vi "Apply Stamp.vi"(8 "error in":errorcluster, 9 "Slot Number":i32, 10 "Chuck Number":i32, 11 "GrabberTool in":refnum<class "GrabberTool Class.lvclass">) -> (0 "error out":errorcluster, 3 "GrabberTool out":refnum<class "GrabberTool Class.lvclass">)   [LabVIEW 2017, in "GrabberTool Class.lvclass"]
uses:
  GrabberTool Class.lvclass
  Config Manager Class/Type Definitions/Part Type.ctl
  Config Manager Class/Type Definitions/Offset.ctl
  WorkTable Class/WorkTable Class.lvclass
  Vec3d Class/Vec3d Class.lvclass
  Config Manager Class/Config Manager Class.lvclass
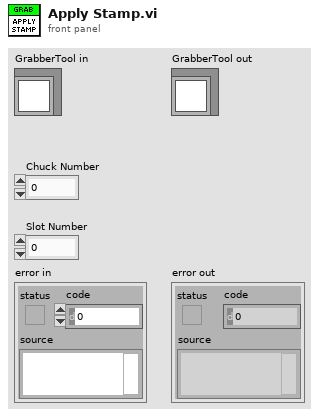
[diagram p1: front panel]
types:
  T1 = enum16{"Empty", "Bare HDI", "Unglued", "Stamped", "PartOnTop", "Weighted", "Unpotted", "Potted"}
  T2 = typedef "Offset.ctl" = enum16{"tool_holder_offset"}
  T3 = typedef "Part Type.ctl" = enum16{"BBM", "HDI", "BARE HDI", "GLUERESERVOIR", "STAMP_1", "STAMP_2", "STAMP_3", "STAMP_4", "STAMP_5", "STAMP_6", "STAMP_7", "STAMP_8", "WEIGHT_1", "WEIGHT_2", "WEIGHT_3", "WEIGHT_4", "WEIGHT_5", "WEIGHT_6", "WEIGHT_7", "WEIGHT_8", "WEIGHT_9", "WEIGHT_10", "WEIGHT_11", "WEIGHT_12", "WEIGHT_13", "WEIGHT_14", "WEIGHT_15", "WEIGHT_16", "PICKER_TOOL", "GRABER_TOOL"}
  T4 = typedef "Worktable_Module Slot.ctl" = cluster{"Slot State":enum16{"Empty", "Bare HDI", "Unglued", "Stamped", "PartOnTop", "Weighted", "Unpotted", "Potted"}, "BBM Type":enum16{"None", "BBM", "GlassSlide"}, "HDI Type":enum16{"None", "HDI", "Polyimide"}, "Vacuum Channel":u8, "Location/Orientation BBM":T5, "Location/Orientation HDI":T5, "S/N":string}
  T5 = typedef "Position_Orientation.ctl" = cluster{"Center":refnum<class "Vec3d Class.lvclass">, "Orientation":refnum<class "Orient3d Class.lvclass">}
  T6 = typedef "Stamp Type.ctl" = enum16{"Stamp 1", "Stamp 2", "Stamp 3", "Stamp 4", "Stamp 5", "Stamp 6", "Stamp 7", "Stamp 8"}
  T7 = typedef "Gluing Parameters.ctl" = cluster{"Safe Grabber Pickup":dbl, "Safe Grabber Lift":dbl, "Glue Resevoir Wait Time":dbl, "Glue BM Wait Time ":dbl, "Placed Weight X-Move":dbl}
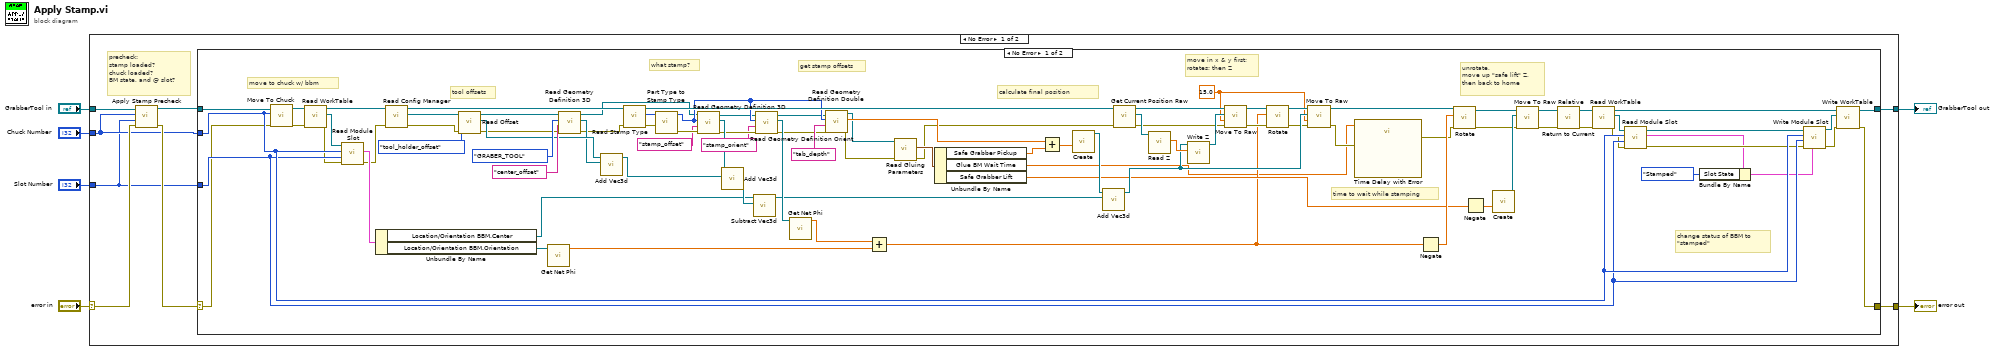
[diagram p0: block diagram]
diagram:
  n1 = case shown="No Error" "error in" {
    selector: "error in" -> [w10 w107]
    tunnel: [w14 w107] -> w6
    tunnel: "GrabberTool in" -> [w12 w108]
    tunnel: [w13 w108] -> w4
    tunnel: "Chuck Number" -> [w8 _]
    tunnel: "Slot Number" -> [w7 _]
    frame No Error {
      # "precheck:\nstamp loaded?\nchuck loaded?\nBM state, and @ slot?"
      n2 = call "Apply Stamp Precheck.vi"("error in (no error)"=w10, "Slot Number"=w7, "Chuck Number"=w8, "GrabberTool Class in"=w12) -> ("error out"=w9:errorcluster, "GrabberTool Class out"=w11:refnum<class "GrabberTool Class.lvclass">)  [unwired: 6 in]
      n3 = case shown="No Error" w9 {
        selector: w9 -> [w44 w106]
        tunnel: [w58 w106] -> w14
        tunnel: [w59 w105] -> w13
        tunnel: w11 -> [w104 w105]
        tunnel: w8 -> [w63 _]
        tunnel: w7 -> [w62 _]
        frame No Error {
          w42 = 15.0 ("Speed")
          # "move to chuck w/ bbm"
          # "time to wait while stamping"
          # "change status of BBM to\n\"stamped\""
          # "unrotate,\nmove up \"safe lift\" Z, \nthen back to home"
          # "move in x & y first;\nrotates; then Z"
          # "calculate final position"
          # "get stamp offsets"
          # "what stamp?"
          # "tool offsets"
          n4 = call-dynamic "Move To Chuck.vi"("error in"=w44, "Chuck"=w63, "Gantry in"=w104) -> ("error out"=w45:errorcluster, "Gantry out"=w101:refnum<class "GrabberTool Class.lvclass">)  [unwired: 7 in]
          n5 = call-dynamic "Read WorkTable.vi"("error in"=w45, "Gantry Class in"=w101) -> ("error out"=w46:errorcluster, "WorkTable Class.lvclass"=w100:refnum<class "WorkTable Class.lvclass">, "Gantry Class out"=w99:refnum<class "GrabberTool Class.lvclass">)  [unwired: 7 in]
          n6 = call-dynamic "Read Module Slot.vi"("error in"=w46, "slot"=w62, "chuck"=w63, "WorkTable in"=w100) -> ("error out"=w47:errorcluster, "Module Slot"=w103:T4)  [unwired: 5 in, 1 out]
          n7 = Unbundle By Name(w103) -> ("Location/Orientation BBM.Center"=w19:refnum<class "Vec3d Class.lvclass">, "Location/Orientation BBM.Orientation"=w89:refnum<class "Orient3d Class.lvclass">)
          n8 = call-dynamic "Read Config Manager.vi"("error in"=w47, "Gantry in"=w99) -> ("error out"=w48:errorcluster, "Config Manager"=w98:refnum<class "Config Manager Class.lvclass">, "Gantry out"=w94:refnum<class "GrabberTool Class.lvclass">)  [unwired: 7 in]
          n9 = call "Read Offset.vi"("error in"=w48, "Offset"=Offset."tool_holder_offset", "Config Manager in"=w98) -> ("error out"=w49:errorcluster, "Vec3d out"=w91:refnum<class "Vec3d Class.lvclass">, "Config Manager out"=w95:refnum<class "Config Manager Class.lvclass">)  [unwired: 6 in]
          n10 = call "Get Net Phi.vi"("Orient3d"=w89) -> ("phi(deg)"=w30:dbl)  [unwired: 8 in, 2 out]
          n11 = call "Read Geometry Definition 3D.vi"("error in"=w49, "Feature"="center_offset", "Part Type"=Part_Type."GRABER_TOOL", "Config Manager in"=w95) -> ("error out"=w50:errorcluster, "Feature Coordinates"=w90:refnum<class "Vec3d Class.lvclass">, "Config Manager out"=w36:refnum<class "Config Manager Class.lvclass">)  [unwired: 5 in]
          n12 = call-dynamic "Add Vec3d.vi"(10:"Vec3d Class in"=w90, 11:"Vec3d Class in"=w91) -> ("Vec3d Class out"=w22:refnum<class "Vec3d Class.lvclass">)  [unwired: 8 in, 1 out]
          n13 = call "Read Stamp Type.vi"("error in (no error)"=w50, "GrabberTool Class in"=w94) -> ("error out"=w51:errorcluster, "Stamp Type"=w93:T6, "GrabberTool Class out"=w83:refnum<class "GrabberTool Class.lvclass">)  [unwired: 7 in]
          n14 = call "Part Type to Stamp Type.vi"("error in"=w51, "Stamp Type"=w93) -> ("error out"=w28:errorcluster, "Part Type"=w37:T3)  [unwired: 8 in]
          n15 = call "Read Geometry Definition 3D.vi"("error in"=w28, "Feature"="stamp_offset", "Part Type"=w37, "Config Manager in"=w36) -> ("error out"=w27:errorcluster, "Feature Coordinates"=w33:refnum<class "Vec3d Class.lvclass">, "Config Manager out"=w35:refnum<class "Config Manager Class.lvclass">)  [unwired: 5 in]
          n16 = call-dynamic "Add Vec3d.vi"(10:"Vec3d Class in"=w22, 11:"Vec3d Class in"=w33) -> ("Vec3d Class out"=w20:refnum<class "Vec3d Class.lvclass">)  [unwired: 8 in, 1 out]
          n17 = call "Subtract Vec3d.vi"("Vec3d in 2"=w20, "Vec3d in 1"=w19) -> ("Vec3d Class out"=w21:refnum<class "Vec3d Class.lvclass">)  [unwired: 8 in, 1 out]
          n18 = call "Read Geometry Definition Orient.vi"("error in"=w27, "Feature"="stamp_orient", "Part Type"=w37, "Config Manager in"=w35) -> ("error out"=w24:errorcluster, "Orient3d out"=w32:refnum<class "Orient3d Class.lvclass">, "Config Manager out"=w34:refnum<class "Config Manager Class.lvclass">)  [unwired: 5 in]
          n19 = call "Get Net Phi.vi"("Orient3d"=w32) -> ("phi(deg)"=w29:dbl)  [unwired: 8 in, 2 out]
          n20 = call "Read Geometry Definition Double.vi"("error in"=w24, "Feature"="tab_depth", "Part Type"=w37, "Config Manager in"=w34) -> ("error out"=w38:errorcluster, "Geometry Definition"=w87:dbl, "Config Manager out"=w39:refnum<class "Config Manager Class.lvclass">)  [unwired: 5 in]
          n21 = Add(x=w29, y=w30) -> (x+y=w31:dbl)
          n22 = call "Read Gluing Parameters.vi"("error in (no error)"=w38, "Config Manager Class in"=w39) -> ("error out"=w52:errorcluster, "Gluing Parameters"=w102:T7)  [unwired: 7 in, 1 out]
          n23 = Unbundle By Name(w102) -> ("Safe Grabber Pickup"=w86:dbl, "Glue BM Wait Time"=w16:dbl, "Safe Grabber Lift"=w73:dbl)
          n24 = Add(x=w87, y=w86) -> (x+y=w85:dbl)
          n25 = call "Create.vi"("Z"=w85) -> ("Vec3d Class out"=w84:refnum<class "Vec3d Class.lvclass">)  [unwired: 9 in, 1 out]
          n26 = call-dynamic "Add Vec3d.vi"(10:"Vec3d Class in"=w21, 11:"Vec3d Class in"=w84) -> ("Vec3d Class out"=w76:refnum<class "Vec3d Class.lvclass">)  [unwired: 8 in, 1 out]
          n27 = call-dynamic "Get Current Position Raw.vi"("error in"=w52, "Gantry in"=w83) -> ("error out"=w23:errorcluster, "Vec3d Class out"=w81:refnum<class "Vec3d Class.lvclass">, "Gantry out"=w82:refnum<class "GrabberTool Class.lvclass">)  [unwired: 7 in]
          n28 = call-dynamic "Read Z.vi"("Vec3d Class in"=w81) -> ("Z"=w80:dbl)  [unwired: 8 in, 2 out]
          n29 = call-dynamic "Write Z.vi"("Z"=w80, "Vec3d Class in"=w76) -> ("Vec3d Class out"=w79:refnum<class "Vec3d Class.lvclass">)  [unwired: 8 in, 1 out]
          n30 = call-dynamic "Move To Raw.vi"("error in"=w23, "Speed"=w42, "Destination"=w79, "Gantry in"=w82) -> ("error out"=w53:errorcluster, "Gantry out"=w78:refnum<class "GrabberTool Class.lvclass">)  [unwired: 6 in]
          n31 = call-dynamic "Rotate.vi"("error in"=w53, "distance(deg)"=w31, "Gantry in"=w78) -> ("error out"=w54:errorcluster, "Gantry out"=w77:refnum<class "GrabberTool Class.lvclass">)  [unwired: 7 in]
          n32 = call-dynamic "Move To Raw.vi"("error in"=w54, "Speed"=w42, "Destination"=w76, "Gantry in"=w77) -> ("error out"=w17:errorcluster, "Gantry out"=w75:refnum<class "GrabberTool Class.lvclass">)  [unwired: 6 in]
          n33 = call "Time Delay with Error.vi"("error in (no error)"=w17, "Delay Time (s)"=w16) -> ("error out"=w15:errorcluster)  [unwired: 9 in]
          n34 = Negate(x=w31) -> (-x=w74:dbl)
          n35 = call-dynamic "Rotate.vi"("error in"=w15, "distance(deg)"=w74, "Gantry in"=w75) -> ("error out"=w69:errorcluster, "Gantry out"=w70:refnum<class "GrabberTool Class.lvclass">)  [unwired: 7 in]
          n36 = Negate(x=w73) -> (-x=w72:dbl)
          n37 = call "Create.vi"("Z"=w72) -> ("Vec3d Class out"=w71:refnum<class "Vec3d Class.lvclass">)  [unwired: 9 in, 1 out]
          n38 = call-dynamic "Move To Raw Relative.vi"("error in"=w69, "Delta"=w71, "Gantry in"=w70) -> ("error out"=w67:errorcluster, "Gantry out"=w68:refnum<class "GrabberTool Class.lvclass">)  [unwired: 7 in]
          n39 = call-dynamic "Return to Current.vi"("error in"=w67, "Gantry in"=w68) -> ("error out"=w65:errorcluster, "Gantry out"=w66:refnum<class "GrabberTool Class.lvclass">)  [unwired: 8 in]
          n40 = call-dynamic "Read WorkTable.vi"("error in"=w65, "Gantry Class in"=w66) -> ("error out"=w55:errorcluster, "WorkTable Class.lvclass"=w64:refnum<class "WorkTable Class.lvclass">, "Gantry Class out"=w61:refnum<class "GrabberTool Class.lvclass">)  [unwired: 7 in]
          n41 = call-dynamic "Read Module Slot.vi"("error in"=w55, "slot"=w62, "chuck"=w63, "WorkTable in"=w64) -> ("error out"=w56:errorcluster, "Module Slot"=w41:T4, "WorkTable out"=w43:refnum<class "WorkTable Class.lvclass">)  [unwired: 5 in]
          n42 = Bundle By Name(cluster=w41, "Slot State"=T1."Stamped") -> (w40:T4)
          n43 = call-dynamic "Write Module Slot.vi"("Module Slot"=w40, "error in"=w56, "slot"=w62, "chuck"=w63, "WorkTable in"=w43) -> ("error out"=w57:errorcluster, "WorkTable out"=w60:refnum<class "WorkTable Class.lvclass">)  [unwired: 5 in]
          n44 = call-dynamic "Write WorkTable.vi"("error in (no error)"=w57, "WorkTable Class.lvclass"=w60, "Gantry Class in"=w61) -> ("error out"=w58:errorcluster, "Gantry Class out"=w59:refnum<class "GrabberTool Class.lvclass">)  [unwired: 7 in]
        }
        frame Error {
        }
      }
    }
    frame Error {
    }
  }
  "error out" <- w6
  "GrabberTool out" <- w4
